vi "set group property caen.vi"(0 "VISA in":refnum<visa-resource-name>, 5 "Group":string, 7 "Property":T1, 9 "Value to set":dbl min=0.0 max=1.0 step=1e-08 format="%.3pA", 11 "error in":errorcluster) -> (4 "VISA out":refnum<visa-resource-name>, 6 "resulting string":string, 15 "error out":errorcluster)   [LabVIEW 2018]
uses:
  Group Properties.ctl
  CAEN globals.vi
panel:
  # "value should be in \nA for current max:\ntype uA or mA"
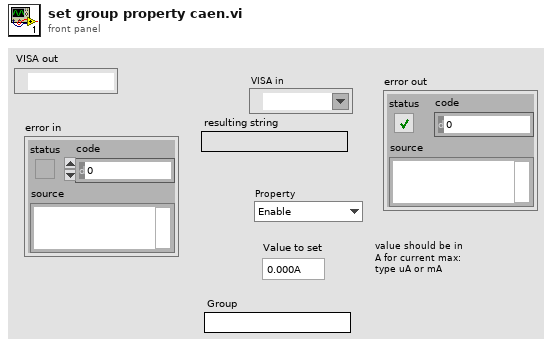
[diagram p1: front panel]
types:
  T1 = typedef "Group Properties.ctl" = enum16{"Enable", "Vset", "Imax", "Vswmax", "Trip Time"}
  T2 = typedef "location cluster.ctl" = cluster{"Column":i32, "Card Type":string, "Channel":i32, "Card":i32, "Default response":string, "Entering":string, "Entering state":bool, "subpage":i32, "page":i32, "Crate":i32, "Screen":string, "Group":string, "Global HV Enable":bool, "Vsel_buffer":bool, "Vdisp_buffer":bool}
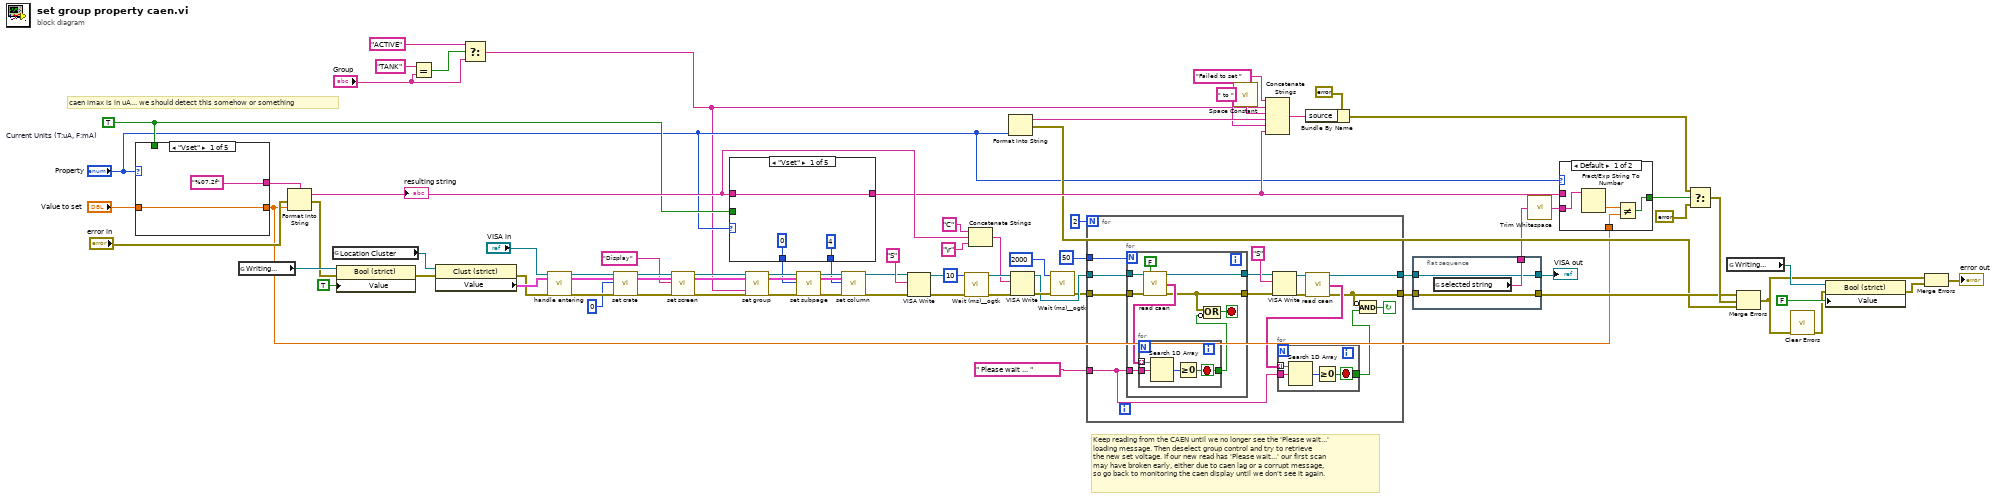
[diagram p0: block diagram]
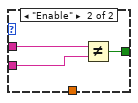
[diagram p2: hidden frame]
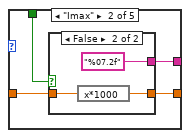
[diagram p3: hidden frame]
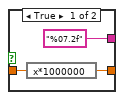
[diagram p4: hidden frame]
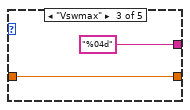
[diagram p5: hidden frame]
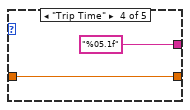
[diagram p6: hidden frame]
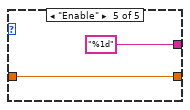
[diagram p7: hidden frame]
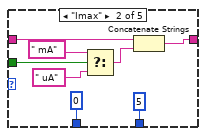
[diagram p8: hidden frame]
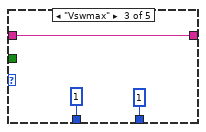
[diagram p9: hidden frame]
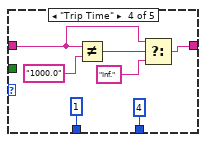
[diagram p10: hidden frame]
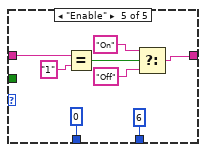
[diagram p11: hidden frame]
diagram:
  w22 = TRUE  # Current Units (T:uA, F:mA)
  # "Keep reading from the CAEN until we no longer see the 'Please wait...' \nloading message. Then deselect group control and try to retrieve\nthe new set voltage. If our new read has 'Please wait...' our first scan\nmay have broken early, either due to caen lag or a corrupt message,\nso go back to monitoring the caen display until we don't see it again."
  # "caen imax is in uA... we should detect this somehow or something"
  n1 = case shown="\"Vset\"" "Property" {
    tunnel: w22 -> [_ w86 _ _ _]
    tunnel: ["%07.2f" w83 "%04d" "%05.1f" "%1d"] -> w35
    tunnel: "Value to set" -> [w81 w85 w93 w95 w98]
    tunnel: [w81 w84 w93 w95 w98] -> w10
    frame "Vset" {
    }
    frame "Imax" {
      n2 = case shown="False" w86 {
        tunnel: [w88 w90] -> w84
        tunnel: w85 -> [w89 w91]
        tunnel: ["%07.2f" "%07.2f"] -> w83
        frame True {
          n3 = expression code="x*1000000"(w89) -> (w88:dbl)
        }
        frame False {
          n4 = expression code="x*1000"(w91) -> (w90:dbl)
        }
      }
    }
    frame "Vswmax" {
    }
    frame "Trip Time" {
    }
    frame "Enable" {
    }
  }
  n5 = global read "CAEN globals.vi" "Writing..."() -> (w76:refnum<vi>)
  n6 = Format Into String(format string=w35, error in="error in", w10) -> (resulting string=w25:string, error out=w18:errorcluster)  [unwired: 1 in]
  "resulting string" <- w25
  n7 = global read "CAEN globals.vi" "Location Cluster"() -> (w77:refnum<vi>)
  n8 = property class="Bool (strict)"(reference=w76, error in=w18, "Value"=TRUE) -> (error out=w19:errorcluster)  [unwired: 1 out]
  n9 = Equal?(x="TANK", y="Group") -> (x = y?=w16:bool)
  n10 = property class="Clust (strict)"(reference=w77, error in=w19) -> (error out=w36:errorcluster, "Value"=w64:T2)  [unwired: 1 out]
  n11 = Select(t="ACTIVE" ("x"), s=w16, f="Group") -> (s? t:f=w1:string)
  n12 = call "handle entering.vi"("VISA in"="VISA in", "Current location"=w64, "error in"=w36) -> ("VISA out"=w73:refnum<visa-resource-name>, "Location Cluster"=w72:T2, "error out"=w71:errorcluster)  [unwired: 14 in]
  n13 = call "set crate.vi"("VISA in"=w73, "Location Cluster in"=w72, "set crate"=0 ("index"), "error in"=w71) -> ("VISA out"=w70:refnum<visa-resource-name>, "Location Cluster out"=w68:T2, "error out"=w69:errorcluster)  [unwired: 13 in]
  n14 = call "set screen.vi"("VISA in"=w70, "Location Cluster in"=w68, "set Screen"="Display", "error in"=w69) -> ("VISA out"=w67:refnum<visa-resource-name>, "Location Cluster out"=w66:T2, "error out"=w65:errorcluster)  [unwired: 13 in]
  n15 = case shown="\"Vset\"" "Property" {
    tunnel: [0 ("set subpage") 0 ("set subpage") 1 ("set subpage") 1 ("set subpage") 0 ("set subpage")] -> w53
    tunnel: [4 ("set column") 5 ("set column") 1 ("set column") 4 ("set column") 6 ("set column")] -> w52
    tunnel: w25 -> [w99 w107 w110 w113 w125]
    tunnel: [w99 w106 w110 w117 w120] -> w24
    tunnel: w22 -> [_ w105 _ _ _]
    frame "Vset" {
    }
    frame "Imax" {
      n16 = Select(t=" mA" ("string"), s=w105, f=" uA" ("string")) -> (s? t:f=w104:string)
      n17 = Concatenate Strings(w107, w104) -> (w106:string)
    }
    frame "Vswmax" {
    }
    frame "Trip Time" {
      n18 = Not Equal?(x=w113, y="1000.0" ("string")) -> (x != y?=w116:bool)
      n19 = Select(t=w113, s=w116, f="Inf." ("string")) -> (s? t:f=w117:string)
    }
    frame "Enable" {
      n20 = Equal?(x=w125, y="1" ("string")) -> (x = y?=w123:bool)
      n21 = Select(t="On" ("string"), s=w123, f="Off" ("string")) -> (s? t:f=w120:string)
    }
  }
  n22 = call "set group.vi"("VISA in"=w67, "Location Cluster in"=w66, "Group"=w1, "error in (no error)"=w65) -> ("VISA out"=w56:refnum<visa-resource-name>, "Location Cluster out"=w55:T2, "error out"=w54:errorcluster)  [unwired: 13 in]
  n23 = call "set subpage.vi"("VISA in"=w56, "Location Cluster in"=w55, "set subpage"=w53, "error in"=w54) -> ("VISA out"=w59:refnum<visa-resource-name>, "Location Cluster out"=w57:T2, "error out"=w58:errorcluster)  [unwired: 13 in]
  n24 = call "set column.vi"("VISA in"=w59, "Location Cluster in"=w57, "set column"=w52, "error in"=w58) -> ("VISA out"=w51:refnum<visa-resource-name>, "error out"=w50:errorcluster)  [unwired: 13 in, 1 out]
  n25 = VISA Write(VISA resource name=w51, write buffer="S" ("string"), error in (no error)=w50) -> (VISA resource name out=w44:refnum<visa-resource-name>, error out=w46:errorcluster)  [unwired: 1 out]
  n26 = call <userlib>:"Wait (ms)__ogtk.vi"("error in (no error)"=w46, "milliseconds to wait"=u32 10) -> ("error out"=w47:errorcluster)  [unwired: 8 in, 1 out]
  n27 = Concatenate Strings("C" ("string"), w25, "\r" ("string")) -> (w43:string)
  n28 = Format Into String("Property") -> (resulting string=w27:string, error out=w23:errorcluster)  [unwired: 3 in]
  n29 = VISA Write(VISA resource name=w44, write buffer=w43, error in (no error)=w47) -> (VISA resource name out=w7:refnum<visa-resource-name>, error out=w42:errorcluster)  [unwired: 1 out]
  n30 = call <userlib>:"Wait (ms)__ogtk.vi"("error in (no error)"=w42, "milliseconds to wait"=u32 2000) -> ("error out"=w6:errorcluster)  [unwired: 8 in, 1 out]
  n31 = for {
    N: 2 -> [_]
    tunnel: 50 -> [w133]
    tunnel: " Please wait ... " ("string") -> [w132]
    tunnel: w7 -> [w137]
    tunnel: [w139] -> w39
    tunnel: w6 -> [w136]
    tunnel: [w130] -> w40
    stop <- w128 continue-if-true
    n32 = for {
      N: w133 -> [_]
      tunnel: w137 -> [w154]
      tunnel: [w152] -> w134
      tunnel: w136 -> [w153]
      tunnel: [w149] -> w135
      tunnel: w132 -> [w146]
      stop <- w147 stop-if-true
      n33 = call "read caen.vi"("VISA in"=w154, "Extended Delay"=FALSE, "error in"=w153) -> ("VISA out"=w152:refnum<visa-resource-name>, "Display array"=w150:string[][], "error out"=w149:errorcluster)  [unwired: 7 in, 3 out]
      n34 = for {
        tunnel: w150 -> [w158] mode=indexing
        tunnel: [w156] -> w148
        tunnel: w146 -> [w155]
        stop <- w156 stop-if-true
        n35 = Search 1D Array(1D array=w158, element=w155) -> (index of element=w157:i32)  [unwired: 1 in]
        n36 = Greater Or Equal To 0?(x=w157) -> (x >= 0?=w156:bool)
      }
      n37 = Compound Arithmetic op=OR(w149, invert w148) -> (w147:bool)
    }
    n38 = VISA Write(VISA resource name=w134, write buffer="S" ("string"), error in (no error)=w135) -> (VISA resource name out=w141:refnum<visa-resource-name>, error out=w140:errorcluster)  [unwired: 1 out]
    n39 = call "read caen.vi"("VISA in"=w141, "error in"=w140) -> ("VISA out"=w139:refnum<visa-resource-name>, "Display array"=w131:string[][], "error out"=w130:errorcluster)  [unwired: 8 in, 3 out]
    n40 = for {
      tunnel: w131 -> [w145] mode=indexing
      tunnel: [w143] -> w129
      tunnel: w132 -> [w142]
      stop <- w143 stop-if-true
      n41 = Search 1D Array(1D array=w145, element=w142) -> (index of element=w144:i32)  [unwired: 1 in]
      n42 = Greater Or Equal To 0?(x=w144) -> (x >= 0?=w143:bool)
    }
    n43 = Compound Arithmetic op=AND(invert w130, w129) -> (w128:bool)
  }
  n44 = call <vilib>:"Space Constant.vi"() -> ("String"=w28:string)
  n45 = Concatenate Strings("Failed to set " ("source"), w1, w28, w27, " to " ("string"), w24) -> (w30:string)
  n46 = Bundle By Name(cluster=errorcluster {"status"=TRUE, "code"=0, "source"="Value not set"} ("error in"), "source"=w30) -> (w32:errorcluster)
  n47 = flat-sequence {
    tunnel: [w161] -> w13
    tunnel: [w160] -> w38
    tunnel: w39 -> [w160]
    tunnel: w40 -> [w159]
    tunnel: [w159] -> w37
    frame #0 {
      n48 = global read "CAEN globals.vi" "selected string"() -> (w161:string)
    }
  }
  n49 = call <vilib>:"Trim Whitespace.vi"("string"=w13) -> ("trimmed string"=w12:string)  [unwired: 1 in]
  n50 = case shown="Default" "Property" {
    tunnel: [w163 w168] -> w80
    tunnel: w12 -> [w162 w166]
    tunnel: w24 -> [_ w167]
    tunnel: w10 -> [w164 _]
    frame Default {
      n51 = Fract/Exp String To Number(string=w162) -> (number=w165:dbl)  [unwired: 3 in, 1 out]
      n52 = Not Equal?(x=w165, y=w164) -> (x != y?=w163:bool)
    }
    frame "Enable" {
      n53 = Not Equal?(x=w167, y=w166) -> (x != y?=w168:bool)
    }
  }
  n54 = Select(t=w32, s=w80, f=errorcluster {"status"=FALSE, "code"=0, "source"=""} ("error in")) -> (s? t:f=w78:errorcluster)
  n55 = global read "CAEN globals.vi" "Writing..."() -> (w20:refnum<vi>)
  n56 = Merge Errors(w37, w78, w23) -> (w9:errorcluster)
  n57 = call <vilib>:"Clear Errors.vi"("error in (no error)"=w9) -> ("error out"=w8:errorcluster)  [unwired: 5 in, 1 out]
  n58 = property class="Bool (strict)"(reference=w20, error in=w8, "Value"=FALSE) -> (error out=w34:errorcluster)  [unwired: 1 out]
  n59 = Merge Errors(w9, w34) -> (→"error out":errorcluster)
  "VISA out" <- w38
